vi "Read Can be inherited.vi"(8 "error in (no error)":errorcluster, 11 "Attribute in":refnum<class "Attribute.lvclass">) -> (0 "error out":errorcluster, 2 "Can be inherited":bool, 3 "Attribute out":refnum<class "Attribute.lvclass">)   [LabVIEW 2021, in "smo.lvlib" / "Attribute.lvclass"]
uses:
  Attribute.lvclass
  Attribute.lvclass/Attribute.ctl
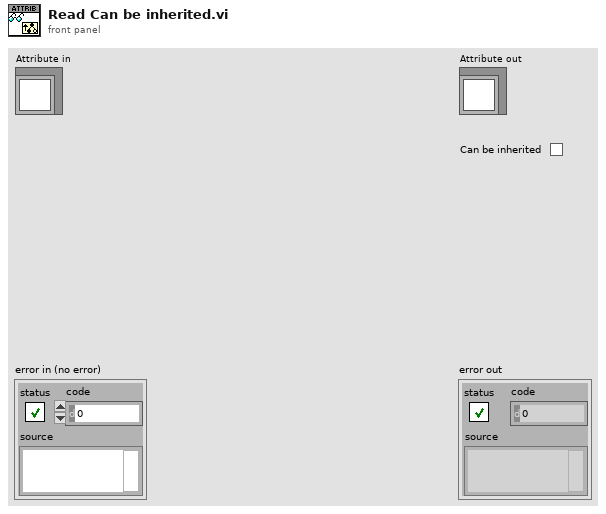
[diagram p1: front panel]
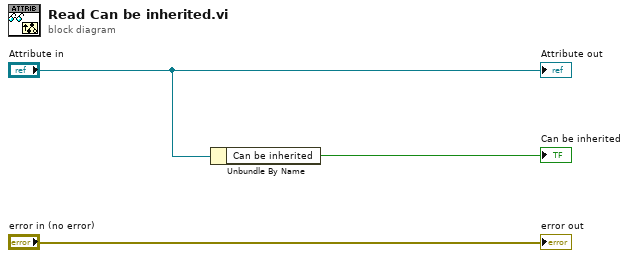
[diagram p0: block diagram]
diagram:
  n1 = Unbundle By Name("Attribute in") -> ("Can be inherited"=→"Can be inherited":bool)
  "error out" <- "error in (no error)"
  "Attribute out" <- "Attribute in"
